vi "saveDataNodeEnd.vi"(8 "error in (no error)":errorcluster, 9 "indent":i32, 10 "XML Refnum in":refnum<file>, 11 "Parameter in":refnum<class "Parameter.lvclass">) -> (0 "error out":errorcluster, 2 "XML Refnum out":refnum<file>, 3 "Parameter out":refnum<class "Parameter.lvclass">)   [LabVIEW 2013, in "Parameter.lvclass"]
doc: "Ends the process of saving a xceData Node to an XML formatted file."
uses:
  Parameter.lvclass
  channel_dataType.ctl
  Parameter.lvclass/Parameter.ctl
panel:
  in  "Data Type":T1
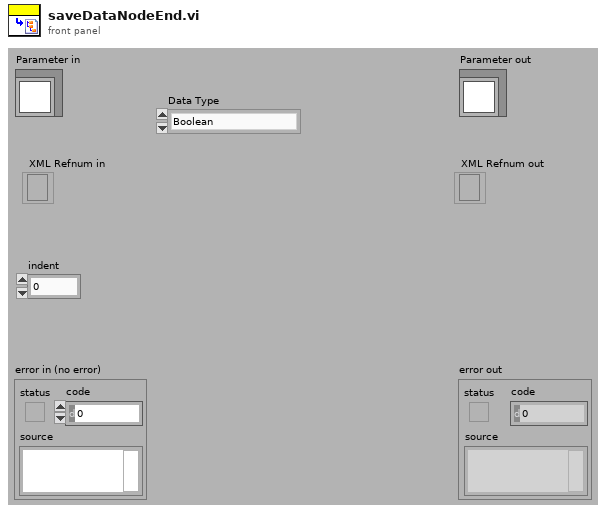
[diagram p1: front panel]
types:
  T1 = typedef "Parameter.lvclass/channel_dataType.ctl" = enum16{"Boolean", "U8", "I8", "U16", "I16", "U32", "I32", "U64", "I64", "FXPI32", "FXPU32", "FXPI64", "FXPU64", "PWM"}
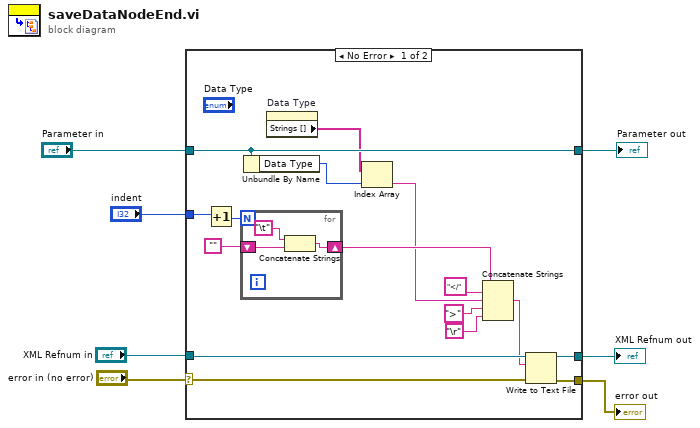
[diagram p0: block diagram]
diagram:
  n1 = case shown="No Error" "error in (no error)" {
    selector: "error in (no error)" -> [w15 w27]
    tunnel: "indent" -> [w8 _]
    tunnel: "XML Refnum in" -> [w18 w28]
    tunnel: "Parameter in" -> [w22 w29]
    tunnel: [w22 w29] -> w3
    tunnel: [w16 w28] -> w2
    tunnel: [w14 w27] -> w1
    frame No Error {
      n2 = Increment(x=w8) -> (x+1=w9:i32)
      n3 = for {
        N: w9 -> [_]
        shift-right: [w26] -> w13
        shift-left: "" -> [w25]
        n4 = Concatenate Strings("\t", w25) -> (w26:string)
      }
      n5 = Unbundle By Name(w22) -> ("Data Type"=w11:T1)
      n6 = property on="Data Type" class="Enum (strict)"() -> ("Strings []"=w12:string[])  [unwired: 2 in, 2 out]
      n7 = Index Array(array=w12, index=w11) -> (element=w10:string)
      n8 = Concatenate Strings(w13, "</", w10, ">", "\r") -> (w17:string)
      n9 = Write to Text File(file (use dialog)=w18, text=w17, error in=w15) -> (refnum out=w16:refnum<file>, error out=w14:errorcluster)  [unwired: 1 in, 1 out]
    }
    frame Error {
    }
  }
  "error out" <- w1
  "Parameter out" <- w3
  "XML Refnum out" <- w2
